vi "ControlPageSelected.vi"(7 "PageSelected":T1(ring), 8 "SolicitudesRecientes":refnum<vi>, 9 "CreditoPyme":refnum<vi>, 10 "PersonaFisica":refnum<vi>, 11 "PersonaMoral":refnum<vi>) -> ()   [LabVIEW 2018]
doc: "Hace el control de animacion de las paginas seleccionadas"
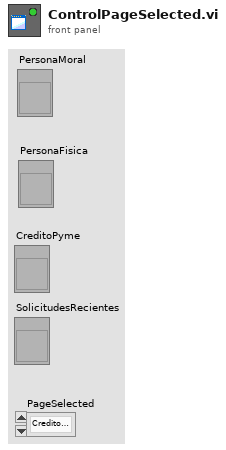
[diagram p1: front panel]
types:
  T1 = enum16{"CreditoPyme", "SolicitudeRecientes", "PersonaFisica", "PersonaMoral"}
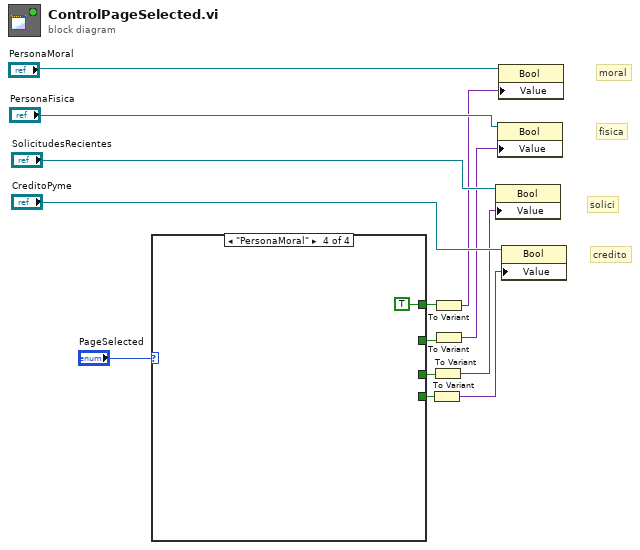
[diagram p0: block diagram]
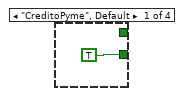
[diagram p2: hidden frame]
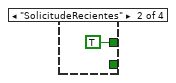
[diagram p3: hidden frame]
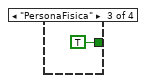
[diagram p4: hidden frame]
diagram:
  # "moral"
  # "fisica"
  # "solici"
  # "credito"
  n1 = case shown="\"PersonaMoral\"" "PageSelected" {
    tunnel: [_ _ _ TRUE] -> w8
    tunnel: [_ _ TRUE _] -> w6
    tunnel: [_ TRUE _ _] -> w5
    tunnel: [TRUE _ _ _] -> w7
    frame "CreditoPyme", Default {
    }
    frame "SolicitudeRecientes" {
    }
    frame "PersonaFisica" {
    }
    frame "PersonaMoral" {
    }
  }
  n2 = To Variant(anything=w7) -> (Variant=w1:variant)
  n3 = To Variant(anything=w5) -> (Variant=w2:variant)
  n4 = To Variant(anything=w8) -> (Variant=w4:variant)
  n5 = To Variant(anything=w6) -> (Variant=w3:variant)
  n6 = property class="Bool"(reference="SolicitudesRecientes", "Value"=w2) -> ()  [unwired: 1 in, 2 out]
  n7 = property class="Bool"(reference="PersonaFisica", "Value"=w3) -> ()  [unwired: 1 in, 2 out]
  n8 = property class="Bool"(reference="PersonaMoral", "Value"=w4) -> ()  [unwired: 1 in, 2 out]
  n9 = property class="Bool"(reference="CreditoPyme", "Value"=w1) -> ()  [unwired: 1 in, 2 out]
